vi "Read equinoxPrefix.vi"(8 "error in (no error)":errorcluster, 11 "RADecParameters in":refnum<class "RADecParameters.lvclass">) -> (0 "error out":errorcluster, 2 "equinoxPrefix":T1, 3 "RADecParameters out":refnum<class "RADecParameters.lvclass">)   [LabVIEW 2014, in "TCSDataDefinitions.lvlib" / "TCSCommand.lvlib" / "TargetConfiguration.lvlib" / "Target.lvlib" / "FixedTarget.lvlib" / "RADecParameters.lvclass"]
uses:
  RADecParameters.lvclass
  Enumerations/EquinoxPrefix.ctl
  RADecParameters.lvclass/RADecParameters.ctl
  FixedTarget.lvlib
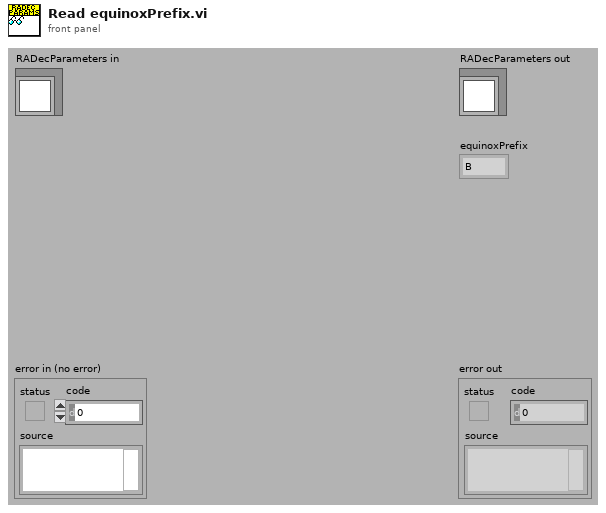
[diagram p1: front panel]
types:
  T1 = typedef "TCSDataDefinitions.lvlib/TCSCommand.lvlib/TargetConfiguration.lvlib/Target.lvlib/FixedTarget.lvlib/EquinoxPrefix.ctl" = enum16{"B", "J"}
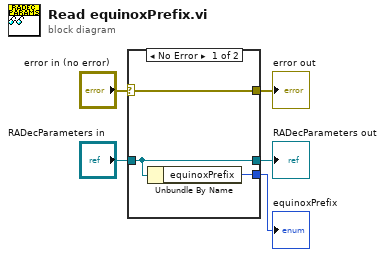
[diagram p0: block diagram]
diagram:
  n1 = case shown="No Error" "error in (no error)" {
    selector: "error in (no error)" -> [w8 w9]
    tunnel: [w8 w9] -> w4
    tunnel: [w7 w10] -> w2
    tunnel: "RADecParameters in" -> [w7 w10]
    tunnel: [w6 _] -> w1
    frame No Error {
      n2 = Unbundle By Name(w7) -> ("equinoxPrefix"=w6:T1)
    }
    frame Error {
    }
  }
  "error out" <- w4
  "RADecParameters out" <- w2
  "equinoxPrefix" <- w1
